vi "TSM SSC Digital Configure Termination Mode.vi"(0 "Digital TSM In":T2, 5 "Termination Mode":T1=1202 items=["High Z"=1202, "Active Load"=1200, "Vterm"=1201], 11 "error in":errorcluster) -> (4 "Digital TSM Out":T2, 15 "error out":errorcluster)   [LabVIEW 2019]
doc: "Specifies the behavior of the specified pin(s) and pin group(s) when the pin driver is in a non-drive pin state (L, H, X, V, M, E)."
uses:
  TSM/TSM SSC Digital.ctl
  <vilib>/NI_TestStand_SemiconductorModule/NI_TestStand_Semiconductor_Module.lvlibp/PinMap/Digital Pattern/PinQueryContext/DigitalPatternPinQueryContext.lvclass
  SSC Digital/SSC Digital.ctl
  <instrlib>/niDigital/niDigital.llb/niDigital Termination Mode.ctl
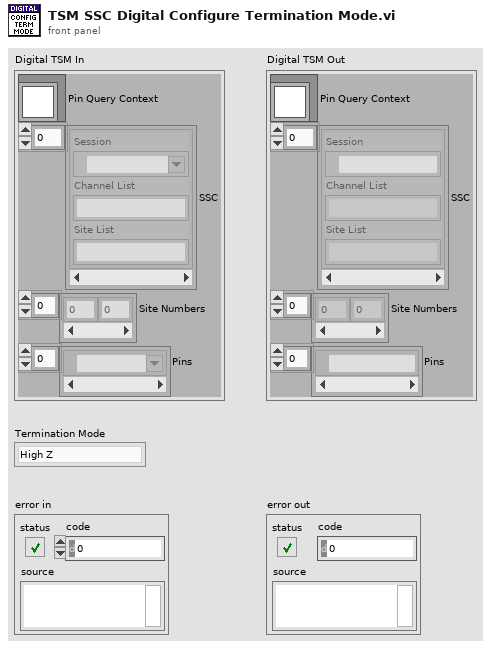
[diagram p1: front panel]
types:
  T1 = typedef "niDigital Termination Mode.ctl" = i32
  T2 = typedef "TSM SSC Digital.ctl" = cluster{"Pin Query Context":refnum<class "DigitalPatternPinQueryContext.lvclass">, "SSC":T3[], "Site Numbers":i32[], "Pins":tag[]}
  T3 = typedef "SSC Digital.ctl" = cluster{"Session":refnum<k15>, "Channel List":string, "Site List":string}
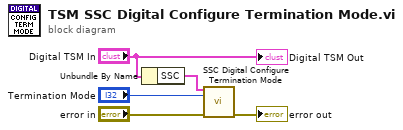
[diagram p0: block diagram]
diagram:
  n1 = Unbundle By Name("Digital TSM In") -> ("SSC"=w4:T3[])
  n2 = call "SSC Digital Configure Termination Mode.vi"("Digital SSC in"=w4, "Termination Mode"="Termination Mode", "error in"="error in") -> ("error out"=→"error out":errorcluster)  [unwired: 11 in, 1 out]
  "Digital TSM Out" <- "Digital TSM In"
